vi "test2Dinter.vi"() -> ()   [LabVIEW 2011]
uses:
  finalCalibTypdef.ctl
  <vilib>/gmath/interp.llb/Interpolate 2D (2d X,Y).vi
  <vilib>/Analysis/8numeric.llb/1D Numeric Integration.vi
  <vilib>/Analysis/NI_AALBase.lvlib
  <vilib>/Analysis/1siggen.llb/Ramp Pattern by Samples.vi
  <vilib>/Analysis/NI_AALPro.lvlib
  <vilib>/gmath/NI_Gmath.lvlib
panel:
  out "subarray":dbl[](graph)
  out "time: 2Dinter":u32=126
  out "time: prepare arrays":u32
  in  "final":T1={"X"=array140x256[35840 elements], "xi"=array140x69[9660 elements], "delta momentum"=0.5, "Y"=array92x256[23552 elements], "yi"=array140x69[9660 elements], "angle (Y)"=[-3.7480215406122, -3.6980215406122, -3.6480215406122, -3.5980215406122, -3.5480215406121998, -3.4980215406122, -3.4480215406122, -3.3980215406122, -3.3480215406122, -3.2980215406121998, -3.2480215406122, -3.1980215406122, -3.1480215406122, -3.0980215406122, -3.0480215406121998, -2.9980215406122, -2.9480215406122, -2.8980215406122, -2.8480215406122, -2.7980215406121998, -2.7480215406122, -2.6980215406122, -2.6480215406122, -2.5980215406121996, -2.5480215406121998, -2.4980215406122, -2.4480215406122, -2.3980215406122, -2.3480215406121996, -2.2980215406121998, -2.2480215406122, -2.1980215406122, -2.1480215406122, -2.0980215406121996, -2.0480215406121998, -1.9980215406122, -1.9480215406122, -1.8980215406121999, -1.8480215406121998, -1.7980215406121998, -1.7480215406122, -1.6980215406121997, -1.6480215406121999, -1.5980215406122, -1.5480215406121998, -1.4980215406122, -1.4480215406121997, -1.3980215406121999, -1.3480215406121996, -1.2980215406121998, -1.2480215406122, -1.1980215406121997, -1.1480215406121999, -1.0980215406121996, -1.0480215406121998, -0.9980215406121999, -0.9480215406121997, -0.8980215406121999, -0.8480215406121996, -0.7980215406121998, -0.7480215406121999, -0.6980215406121997, -0.6480215406121999, -0.5980215406121996, -0.5480215406121998, -0.49802154061219994, -0.4480215406121997, -0.39802154061219985, -0.3480215406121996, -0.29802154061219976, -0.24802154061219994, -0.19802154061219968, -0.14802154061219985, -0.09802154061219959, -0.048021540612199765, 0.001978459387800058, 0.051978459387800324, 0.10197845938780015, 0.1519784593878004, 0.20197845938780024, 0.25197845938780006, 0.3019784593877999, 0.3519784593878006, 0.4019784593878004, 0.45197845938780024, 0.5019784593878001, 0.5519784593877999, 0.6019784593878006, 0.6519784593878004, 0.7019784593878002, 0.7519784593878001, 0.8019784593877999, 0.8519784593878006, 0.9019784593878004, 0.9519784593878002, 1.0019784593878, 1.0519784593878008, 1.1019784593878006, 1.1519784593878004, 1.2019784593878002, 1.2519784593878, 1.3019784593878008, 1.3519784593878006, 1.4019784593878004, 1.4519784593878002, 1.5019784593878, 1.5519784593878008, 1.6019784593878006, 1.6519784593878004, 1.7019784593878002, 1.7519784593878, 1.8019784593878008, 1.8519784593878006, 1.9019784593878004, 1.9519784593878002, 2.0019784593878, 2.0519784593878008, 2.1019784593878006, 2.1519784593878004, 2.2019784593878002, 2.2519784593878, 2.3019784593878008, 2.3519784593878006, 2.4019784593878004, 2.4519784593878002, 2.5019784593878, 2.5519784593878008, 2.6019784593878006, 2.6519784593878004, 2.7019784593878002, 2.7519784593878, 2.8019784593878008, 2.8519784593878006, 2.9019784593878004, 2.9519784593878002, 3.0019784593878, 3.0519784593878008, 3.1019784593878006, 3.1519784593878004, 3.2019784593878002], "delta angle"=0.04999999999999982, "scale delta angle"=1.3341308871728326, "intraX"=69.0, "intraY"=140.0, "mask"=array140x69[9660 elements]}
  in  "Y angles 2D":dbl[][](graph)=array92x256[23552 elements]
  in  "Momentum [MeV/C]":dbl[](graph)=[50.07229753265274, 50.15983071443298, 50.24744305307639, 50.335473133793386, 50.42362482327455, 50.512110383361254, 50.60080468664528, 50.68974523698868, 50.77898610800287, 50.86838180578416, 50.95817657226504, 51.04807238565412, 51.138390361009556, 51.22885558514154, 51.31963681309364, 51.41067480417576, 51.50191835219721, 51.593533353084716, 51.68526688034519, 51.777441364408986, 51.869765957355305, 51.962407630762286, 52.05532861013082, 52.148440323478574, 52.24196272933561, 52.33562113373428, 52.429670064721215, 52.52393805106378, 52.61845821707546, 52.71334325025615, 52.8083776798975, 52.90384554844539, 52.999508499681035, 53.09545010289294, 53.19174647851, 53.28820539308308, 53.38510251597625, 53.48220608299536, 53.579579491932385, 53.677325478650495, 53.77524407497087, 53.87356454114524, 53.97213509708919, 54.07092947555539, 54.17015652080565, 54.269570248674576, 54.36932324018744, 54.46941123347271, 54.56969420713886, 54.67041102722302, 54.77137308543024, 54.87257300044643, 54.974216610337685, 55.07606355335658, 55.178218731599664, 55.28075162708607, 55.383497615374985, 55.48661882716664, 55.59006868597277, 55.69374082051916, 55.79784018182734, 55.90223156342043, 56.00684549505606, 56.111873606754635, 56.21720302119806, 56.32283918208316, 56.42882890219444, 56.5351236728704, 56.641720134138744, 56.748684625045605, 56.855953718041384, 56.963538804395505, 57.07149018048698, 57.1797524193871, 57.28834570048473, 57.397296090985385, 57.50656005590199, 57.616172858663234, 57.7261282182496, 57.83640050845812, 57.94704953896948, 58.05802395807821, 58.16933872771148, 58.281018950382276, 58.393019385067475, 58.50539236287636, 58.61810188547397, 58.731156613509306, 58.844584735455136, 58.95833890016895, 59.07248879093084, 59.18696647546072, 59.30181925309975, 59.417024114353715, 59.53258299516336, 59.64851910190262, 59.76479881890396, 59.88148018668999, 59.9984946345451, 60.115921847826904, 60.23368516435314, 60.35185067203749, 60.470364539014994, 60.58927639342781, 60.70854834588829, 60.8282217835343, 60.94825921065038, 61.06870460119095, 61.18951111605114, 61.310724517923916, 61.43229968923823, 61.554292936903096, 61.67664895324813, 61.799436232216266, 61.922589641352786, 62.04618162330728, 62.17014251711384, 62.29452558712144, 62.41929351908275, 62.54446961953862, 62.67006038580525, 62.7960388070786, 62.92246671292553, 63.04927783564081, 63.176524732148735, 63.304179330384684, 63.43223718780839, 63.560740627474246, 63.689640295677854, 63.81898202265973, 63.94874959300494, 64.07892098001717, 64.20955602995856, 64.34059773887691, 64.47206231218102, 64.60397897467172, 64.73631237640821, 64.869085738597, 65.00231471477268, 65.13596573408442, 65.27006683532953, 65.40462738222232, 65.53962005497071, 65.67506033230055, 65.8109815987919, 65.9473433427755, 66.0841535752014, 66.22144522937742, 66.35918942385068, 66.49737914455044, 66.63602368841578, 66.7751474034366, 66.91472762039646, 67.05476469204305, 67.19527658421696, 67.33628142329019, 67.47775433008199, 67.61969559362808, 67.76210633768139, 67.90501441704042, 68.04840416594494, 68.19226957401172, 68.33661620544575, 68.48144943209485, 68.62679493465447, 68.77262969523863, 68.91895730915441, 69.06577899650894, 69.21310202770283, 69.36092815635924, 69.50927035473094, 69.65811068326026, 69.80744438410392, 69.9572688425338, 70.10759120897865, 70.25841815946569, 70.4097512757638, 70.56160058811538, 70.71397754166274, 70.86686942159963, 71.02027152856012, 71.17418729848787, 71.32861278943483, 71.48355948930313, 71.63903383298718, 71.79503909451408, 71.95157896275194, 72.10865976498366, 72.26627835863347, 72.42443773423045, 72.58313719524446, 72.74237809740015, 72.90216284371118, 73.06249307935462, 73.22337570366312, 73.38481299401033, 73.54681679847542, 73.70938657108235, 73.87252626016662, 74.03623956556689, 74.20052907315498, 74.36539661252398, 74.53084771684584, 74.6968830777154, 74.86350384169735, 75.03070688990859, 75.19849228216307, 75.36687898015636, 75.53585900252442, 75.70544362170186, 75.87563942077512, 76.04645285122083, 76.21787961399053, 76.38991264403143, 76.56255744104838, 76.73582111277462, 76.9096873341793, 77.08416070831274, 77.25925052021022, 77.4349600453981, 77.6113063980163, 77.78827696200767, 77.9658595260864, 78.14405451011176, 78.32286883536608, 78.50233423633921, 78.68243479312856, 78.8631773205512, 79.0445771403343, 79.22665527344569, 79.40938326412468, 79.59275150859004, 79.77678280996797, 79.96146342460078, 80.14678490571335, 80.3327747387059, 80.51944409828232, 80.70678449184061, 80.89483312815786, 81.08358530541098, 81.27300980796292, 81.463137571359, 81.65394598409715, 81.84543408487188, 82.03763762101902, 82.23053281769182, 82.42416900544262, 82.61852659219059, 82.81361926820861, 83.00944812670377, 83.20598132803654, 83.40325366033011, 83.6012275391606, 83.79997131222892, 83.99943721084946, 84.19970193525548]
  in  "pixel angle (y)":dbl[](array[numeric])=[0.037477582207811125, 0.0375378103280183, 0.03759835324988168, 0.037638239676906486, 0.03767220925926772, 0.037689747456214555, 0.037718124937573545, 0.037759339175450615, 0.037815945617947995, 0.03788063743518453, 0.037925600705336834, 0.03796557132360937, 0.0379840699612592, 0.03800781476200766, 0.03804282848571206, 0.03808205383420604, 0.038124687047283425, 0.03819497257668394, 0.03827047431284569, 0.03831511839702091, 0.03834959008082911, 0.038362398521621585, 0.03839429519350118, 0.03843930535194785, 0.038506475559157566, 0.03857307729220705, 0.038620070814944035, 0.03866676181810502, 0.0387130848375811, 0.03873601391808348, 0.03875484132448539, 0.03880297443490419, 0.03886161595012056, 0.03893532872686465, 0.03881951069724796, 0.038611566223731374, 0.038105163864268106, 0.03769554724778958, 0.03740223373517817, 0.03723603496248856, 0.037173529161227875, 0.03749521823198995, 0.03783880798538115, 0.03820360723024477, 0.038739908755063765, 0.03919553366910764, 0.039389798714018424, 0.03953215344479871, 0.03964512210299738, 0.03969861147758047, 0.03976617071201567, 0.03984752086655404, 0.03990445098286168, 0.03995783288040166, 0.04000815111780023, 0.04004296007757376, 0.04007772601145543, 0.04012660954541183, 0.04020430873594673, 0.04029042274207045, 0.040339384000090406, 0.04039344990701764, 0.04044723736216941, 0.040462083471605036, 0.040551826962865384, 0.04057158550151761, 0.04064707182832961, 0.04069310897748229, 0.040726185871045435, 0.0407104047486137, 0.040722698074851925, 0.040790994765831104, 0.040786483184387635, 0.040900331433328066, 0.04100957841477542, 0.04113275717285748, 0.04128943624065327, 0.041383986129591356, 0.04152035652895744, 0.04158841056385747, 0.041693110815272556, 0.04176647471980758, 0.041808109547457964, 0.041896373749087015, 0.041945596201376605, 0.04203752144656966, 0.042096929899642394, 0.04216377175264231, 0.04221267837449374, 0.04225164716353927, 0.04233033219068084, 0.04240479044280577, 0.0424280109007416, 0.04252130522978519, 0.04255646064460216, 0.04262159712046446, 0.04271106684539846, 0.042726953841267706, 0.042834365027920374, 0.04285980067144029, 0.04290407847360533, 0.04298148359330201, 0.043059352930560964, 0.04310666304059418, 0.04318186470763455, 0.04321124753836594, 0.04326638956928416, 0.04336841907624626, 0.043372840226511486, 0.04344502754224136, 0.043458805969808625, 0.04350176453092871, 0.04354504692756502, 0.043572282445234374, 0.043719886246918596, 0.04377506306562891, 0.0438307216429467, 0.043882255177807514, 0.043967069555529224, 0.04404340617312178, 0.044087710081034515, 0.04422154778325681, 0.04424178336968342, 0.04425229311880168, 0.044328392796142854, 0.04440326745130848, 0.04447921973832866, 0.04449440271083517, 0.0445909980356023, 0.04465122004116054, 0.04469582940733911, 0.044746207718220174, 0.044675726002842364, 0.04267205785741442, 0.04276641846475699, 0.04280525728079379, 0.04285689437155202, 0.042923903830319854, 0.04301110520013367, 0.0431323830019876, 0.04316545752017941, 0.04328575986704131, 0.043384775227001564, 0.04349267378173057, 0.04355348288319274, 0.043604651859098995, 0.043716347210854205, 0.04378821118055596, 0.04386448742162739, 0.04399794933329327, 0.04404503831307389, 0.04421272483161148, 0.044331415250278665, 0.04440921929214469, 0.04454672370056835, 0.04460184505873057, 0.04466448019056487, 0.04475018057724128, 0.04484458912204318, 0.044920986274926945, 0.045002289062931904, 0.045097118158317455, 0.04518240711607863, 0.045269624867765396, 0.04541703071251877, 0.04550795280628246, 0.04559946882095624, 0.04571174005768977, 0.0460750366911433, 0.04639562647607986, 0.04674801712470383, 0.04710979552536287, 0.047363521515647794, 0.04741983739378383, 0.04732957065712525, 0.047199255919237446, 0.04702192063132577, 0.04689077900955041, 0.04721790956291122, 0.04754662503244337, 0.04779302473044378, 0.04818681974992477, 0.04858485464933235, 0.04869299591718263, 0.048584550402762744, 0.0484764930169296, 0.04835834443169048, 0.04828719469900186, 0.048222766428404916, 0.04834188706300746, 0.04846143489496384, 0.04857102710814599, 0.04868653104243684, 0.04880619805934796, 0.04893075858982508, 0.04908427889763241, 0.049511031973531044, 0.049898237974339496, 0.05040624016531754, 0.050837732267569075, 0.05134015949012785, 0.0516218346028756, 0.05178360005226867, 0.05194105378254242, 0.05214945752433647, 0.052362654325496354, 0.05255736775078291, 0.05271697114435879, 0.052902655552384936, 0.05345104909708188, 0.05400078856621423, 0.05457402723638789, 0.05525483903273678, 0.05589234596637011, 0.056344461115130355, 0.05660466064617305, 0.05684739692395777, 0.056939091390825536, 0.057216581293874316, 0.05752631629729546, 0.05776594597871566, 0.057970210025959985, 0.05834620444709129, 0.059095734294158916, 0.05966843750713058, 0.060504562685601664, 0.06104390929579467, 0.06184660565948633, 0.06229432111910379, 0.06285675616055271, 0.06335993292100976, 0.0640103781230761, 0.06494640922743135, 0.06537375904368167, 0.06452970332711605, 0.06398947667297139, 0.06318949092368346, 0.06310561739014162, 0.06273982627858529, 0.06317953539335003, 0.064788318139689, 0.0670660575425553, 0.06825261980428583, 0.06928919838614656, 0.07047135756226576, 0.07108681736337749, 0.07212300303227219, 0.07274371033405448, 0.07331974443237226, 0.07396837480214184, 0.07437897672000632, 0.07495723436598267, 0.07528920281146867, 0.07587775203900965, 0.0762276605751895, 0.07649023552269796]
  out "time: spectra":u32=1
  out "spec cluster 2":cluster{"Momentum [MeV/C]":dbl[], dbl[]}(graph)={"Momentum [MeV/C]"=[50.07229753265274, 50.57229753265274, 51.07229753265274, 51.57229753265274, 52.07229753265274, 52.57229753265274, 53.07229753265274, 53.57229753265274, 54.07229753265274, 54.57229753265274, 55.07229753265274, 55.57229753265274, 56.07229753265274, 56.57229753265274, 57.07229753265274, 57.57229753265274, 58.07229753265274, 58.57229753265274, 59.07229753265274, 59.57229753265274, 60.07229753265274, 60.57229753265274, 61.07229753265274, 61.57229753265274, 62.07229753265274, 62.57229753265274, 63.07229753265274, 63.57229753265274, 64.07229753265274, 64.57229753265274, 65.07229753265274, 65.57229753265274, 66.07229753265274, 66.57229753265274, 67.07229753265274, 67.57229753265274, 68.07229753265274, 68.57229753265274, 69.07229753265274, 69.57229753265274, 70.07229753265274, 70.57229753265274, 71.07229753265274, 71.57229753265274, 72.07229753265274, 72.57229753265274, 73.07229753265274, 73.57229753265274, 74.07229753265274, 74.57229753265274, 75.07229753265274, 75.57229753265274, 76.07229753265274, 76.57229753265274, 77.07229753265274, 77.57229753265274, 78.07229753265274, 78.57229753265274, 79.07229753265274, 79.57229753265274, 80.07229753265274, 80.57229753265274, 81.07229753265274, 81.57229753265274, 82.07229753265274, 82.57229753265274, 83.07229753265274, 83.57229753265274, 84.07229753265274], [0.0867981540222726, 0.08261634745549262, 0.15780243233786856, 0.14775796013035777, 0.05263053391121891, 0.053052912294376156, 0.15191318594308015, 0.14981983430136114, 0.11700139206762095, 0.13155222887076734, 0.1684249055215002, 0.16857865833690094, 0.14176424686395364, 0.14427921628046295, 0.1644688231907754, 0.1635416016001087, 0.1420908968440197, 0.14020609014657043, 0.1588669769760078, 0.15589370121820792, 0.14174948409773352, 0.13341276225310042, 0.13536702340099901, 0.14916877693013172, 0.14718055167799698, 0.12846317488550774, 0.12676970679561064, 0.12937916674428734, 0.13973463531757968, 0.13218113303417095, 0.11053750184758489, 0.10576539321438339, 0.10038686906156509, 0.12463763630849774, 0.12106677338062412, 0.12028186596589945, 0.09139884919877436, 0.09412084211729885, 0.12365896282614211, 0.12893346320853483, 0.13058812446128448, 0.10610796495898847, 0.10366759807927937, 0.10497898421031235, 0.12419714648561285, 0.13205036294523848, 0.13253036025692783, 0.1309733623420704, 0.1137779761530524, 0.11728841296657326, 0.12239930144646781, 0.14675371437352117, 0.15014047187903135, 0.15234650208833272, 0.13443316248670253, 0.12377935992042939, 0.12145373556854189, 0.1416095768605585, 0.16143985441865993, 0.1655396857388431, 0.16905287974194014, 0.13483627511386545, 0.12806962985094095, 0.13850098246313058, 0.14688829788141392, 0.18928965954454857, 0.19215368111241415, 0.19521128738469867, 0.20641294822426734]}
  out "charge (spectra)":dbl=4.5665602092068625 format="%0.4f"
  out "charge (YSum)":dbl=4.639584559364366 format="%0.4f"
  out "Sum Y":cluster{"Ramp Pattern":dbl[], dbl[]}={"Ramp Pattern"=[-3.7480215406122, -3.6980215406122, -3.6480215406122, -3.5980215406122, -3.5480215406121998, -3.4980215406122, -3.4480215406122, -3.3980215406122, -3.3480215406122, -3.2980215406121998, -3.2480215406122, -3.1980215406122, -3.1480215406122, -3.0980215406122, -3.0480215406121998, -2.9980215406122, -2.9480215406122, -2.8980215406122, -2.8480215406122, -2.7980215406121998, -2.7480215406122, -2.6980215406122, -2.6480215406122, -2.5980215406121996, -2.5480215406121998, -2.4980215406122, -2.4480215406122, -2.3980215406122, -2.3480215406121996, -2.2980215406121998, -2.2480215406122, -2.1980215406122, -2.1480215406122, -2.0980215406121996, -2.0480215406121998, -1.9980215406122, -1.9480215406122, -1.8980215406121999, -1.8480215406121998, -1.7980215406121998, -1.7480215406122, -1.6980215406121997, -1.6480215406121999, -1.5980215406122, -1.5480215406121998, -1.4980215406122, -1.4480215406121997, -1.3980215406121999, -1.3480215406121996, -1.2980215406121998, -1.2480215406122, -1.1980215406121997, -1.1480215406121999, -1.0980215406121996, -1.0480215406121998, -0.9980215406121999, -0.9480215406121997, -0.8980215406121999, -0.8480215406121996, -0.7980215406121998, -0.7480215406121999, -0.6980215406121997, -0.6480215406121999, -0.5980215406121996, -0.5480215406121998, -0.49802154061219994, -0.4480215406121997, -0.39802154061219985, -0.3480215406121996, -0.29802154061219976, -0.24802154061219994, -0.19802154061219968, -0.14802154061219985, -0.09802154061219959, -0.048021540612199765, 0.001978459387800058, 0.051978459387800324, 0.10197845938780015, 0.1519784593878004, 0.20197845938780024, 0.25197845938780006, 0.3019784593877999, 0.3519784593878006, 0.4019784593878004, 0.45197845938780024, 0.5019784593878001, 0.5519784593877999, 0.6019784593878006, 0.6519784593878004, 0.7019784593878002, 0.7519784593878001, 0.8019784593877999, 0.8519784593878006, 0.9019784593878004, 0.9519784593878002, 1.0019784593878, 1.0519784593878008, 1.1019784593878006, 1.1519784593878004, 1.2019784593878002, 1.2519784593878, 1.3019784593878008, 1.3519784593878006, 1.4019784593878004, 1.4519784593878002, 1.5019784593878, 1.5519784593878008, 1.6019784593878006, 1.6519784593878004, 1.7019784593878002, 1.7519784593878, 1.8019784593878008, 1.8519784593878006, 1.9019784593878004, 1.9519784593878002, 2.0019784593878, 2.0519784593878008, 2.1019784593878006, 2.1519784593878004, 2.2019784593878002, 2.2519784593878, 2.3019784593878008, 2.3519784593878006, 2.4019784593878004, 2.4519784593878002, 2.5019784593878, 2.5519784593878008, 2.6019784593878006, 2.6519784593878004, 2.7019784593878002, 2.7519784593878, 2.8019784593878008, 2.8519784593878006, 2.9019784593878004, 2.9519784593878002, 3.0019784593878, 3.0519784593878008, 3.1019784593878006, 3.1519784593878004, 3.2019784593878002], [0.011137016165256157, 0.021829482575962254, 0.03253936074405018, 0.03253936074405018, 0.04311640649190382, 0.04311640649190382, 0.05396432999147681, 0.05396432999147681, 0.05396432999147681, 0.0648405149308176, 0.0648405149308176, 0.07519709540305819, 0.08532238926169682, 0.10645960013879904, 0.11646552616110853, 0.1262931972965455, 0.1262931972965455, 0.13613073955062374, 0.14616184635933333, 0.1568268520872908, 0.16764674670326793, 0.1792333420896368, 0.1792333420896368, 0.19119255194621682, 0.21580323036808718, 0.22798757479306148, 0.24004934637789171, 0.27425739243614305, 0.2954593954326747, 0.3268444217371545, 0.33699626234794267, 0.3972438893400589, 0.4975079821041705, 0.5784550978937094, 0.6237641671768127, 0.670223308632034, 0.6972386282522536, 0.7194304027948516, 0.7614949581566398, 0.7750502096335162, 0.8081105417562462, 0.8400022408477874, 0.8625280417911433, 0.8842068672698414, 0.9042665147796451, 0.9307604876664245, 1.141986935321149, 1.1459565922804242, 1.1499446962467175, 1.1534926992504548, 1.157688284154065, 1.1602617774340027, 1.1628196339295893, 1.0532823804226565, 1.0068490061377193, 1.0018659739534326, 1.0077449998924777, 1.0106962243007982, 1.0201814437681154, 1.1327018238729718, 1.1841597444446181, 1.1898496190570238, 1.1917683993566488, 1.1944768150871825, 1.197472826548403, 1.196932235338961, 1.1761955574199705, 1.0340587513385475, 1.0326774256268136, 1.0333844213877457, 1.0333800781324616, 1.0365329736868745, 1.0533459332692046, 1.2020056041761717, 1.2060281105825565, 1.2050317606479317, 1.204201827833067, 1.2043812850997597, 1.2046266645753132, 1.1996280056100217, 1.0677778229501242, 1.0209979917006726, 1.0152144652017994, 1.0150612256540354, 1.0176812530801653, 1.024219078901479, 1.150812963763347, 1.2064688058325819, 1.208526307739713, 1.2098977578471666, 1.2103459979931248, 1.2124905744228602, 1.2136908075909367, 1.1858763420838527, 1.0053181621971135, 0.9979875683723081, 0.9933271834735534, 0.9872596918513727, 0.9810110365998367, 0.9985706652221166, 1.2003841515450748, 1.2036401493895261, 1.1982963556918365, 1.1922389934162032, 1.1863304015351999, 1.1669414647412235, 1.1581835128027165, 1.017484351991429, 0.9006904091068436, 0.8586545614337409, 0.7663944573911133, 0.6290660218141425, 0.5007457951411629, 0.4280535100713805, 0.4099891022028317, 0.38164291917095694, 0.29668556124489337, 0.2797331706247183, 0.2715140650224642, 0.26328795499237434, 0.23670749597480242, 0.21926816308825772, 0.21926816308825772, 0.1883408228071427, 0.1707249762001949, 0.1707249762001949, 0.15632749156797304, 0.14855651092515887, 0.12097184081735882, 0.10366193619417946, 0.08636660795112303, 0.08636660795112303, 0.08636660795112303, 0.0784992419374238, 0.0784992419374238, 0.06971613723795841, 0.06971613723795841, 0.03515066658752093, 0.017933506702217872, 0.0]}
  out "Array":dbl[][](array[numeric])
  out "charge (sum)":dbl=4.639862984768497
  out "charge density":dbl[][](array[numeric])
  out "Z 2":dbl[][](graph)
  out "size(s)":i32[](array[numeric])=[140, 69]
  out "size(s) 2":i32[](array[numeric])=[140, 69]
  in  "empty image":bool
  in  "Z":dbl[][](graph)=array92x256[23552 elements]
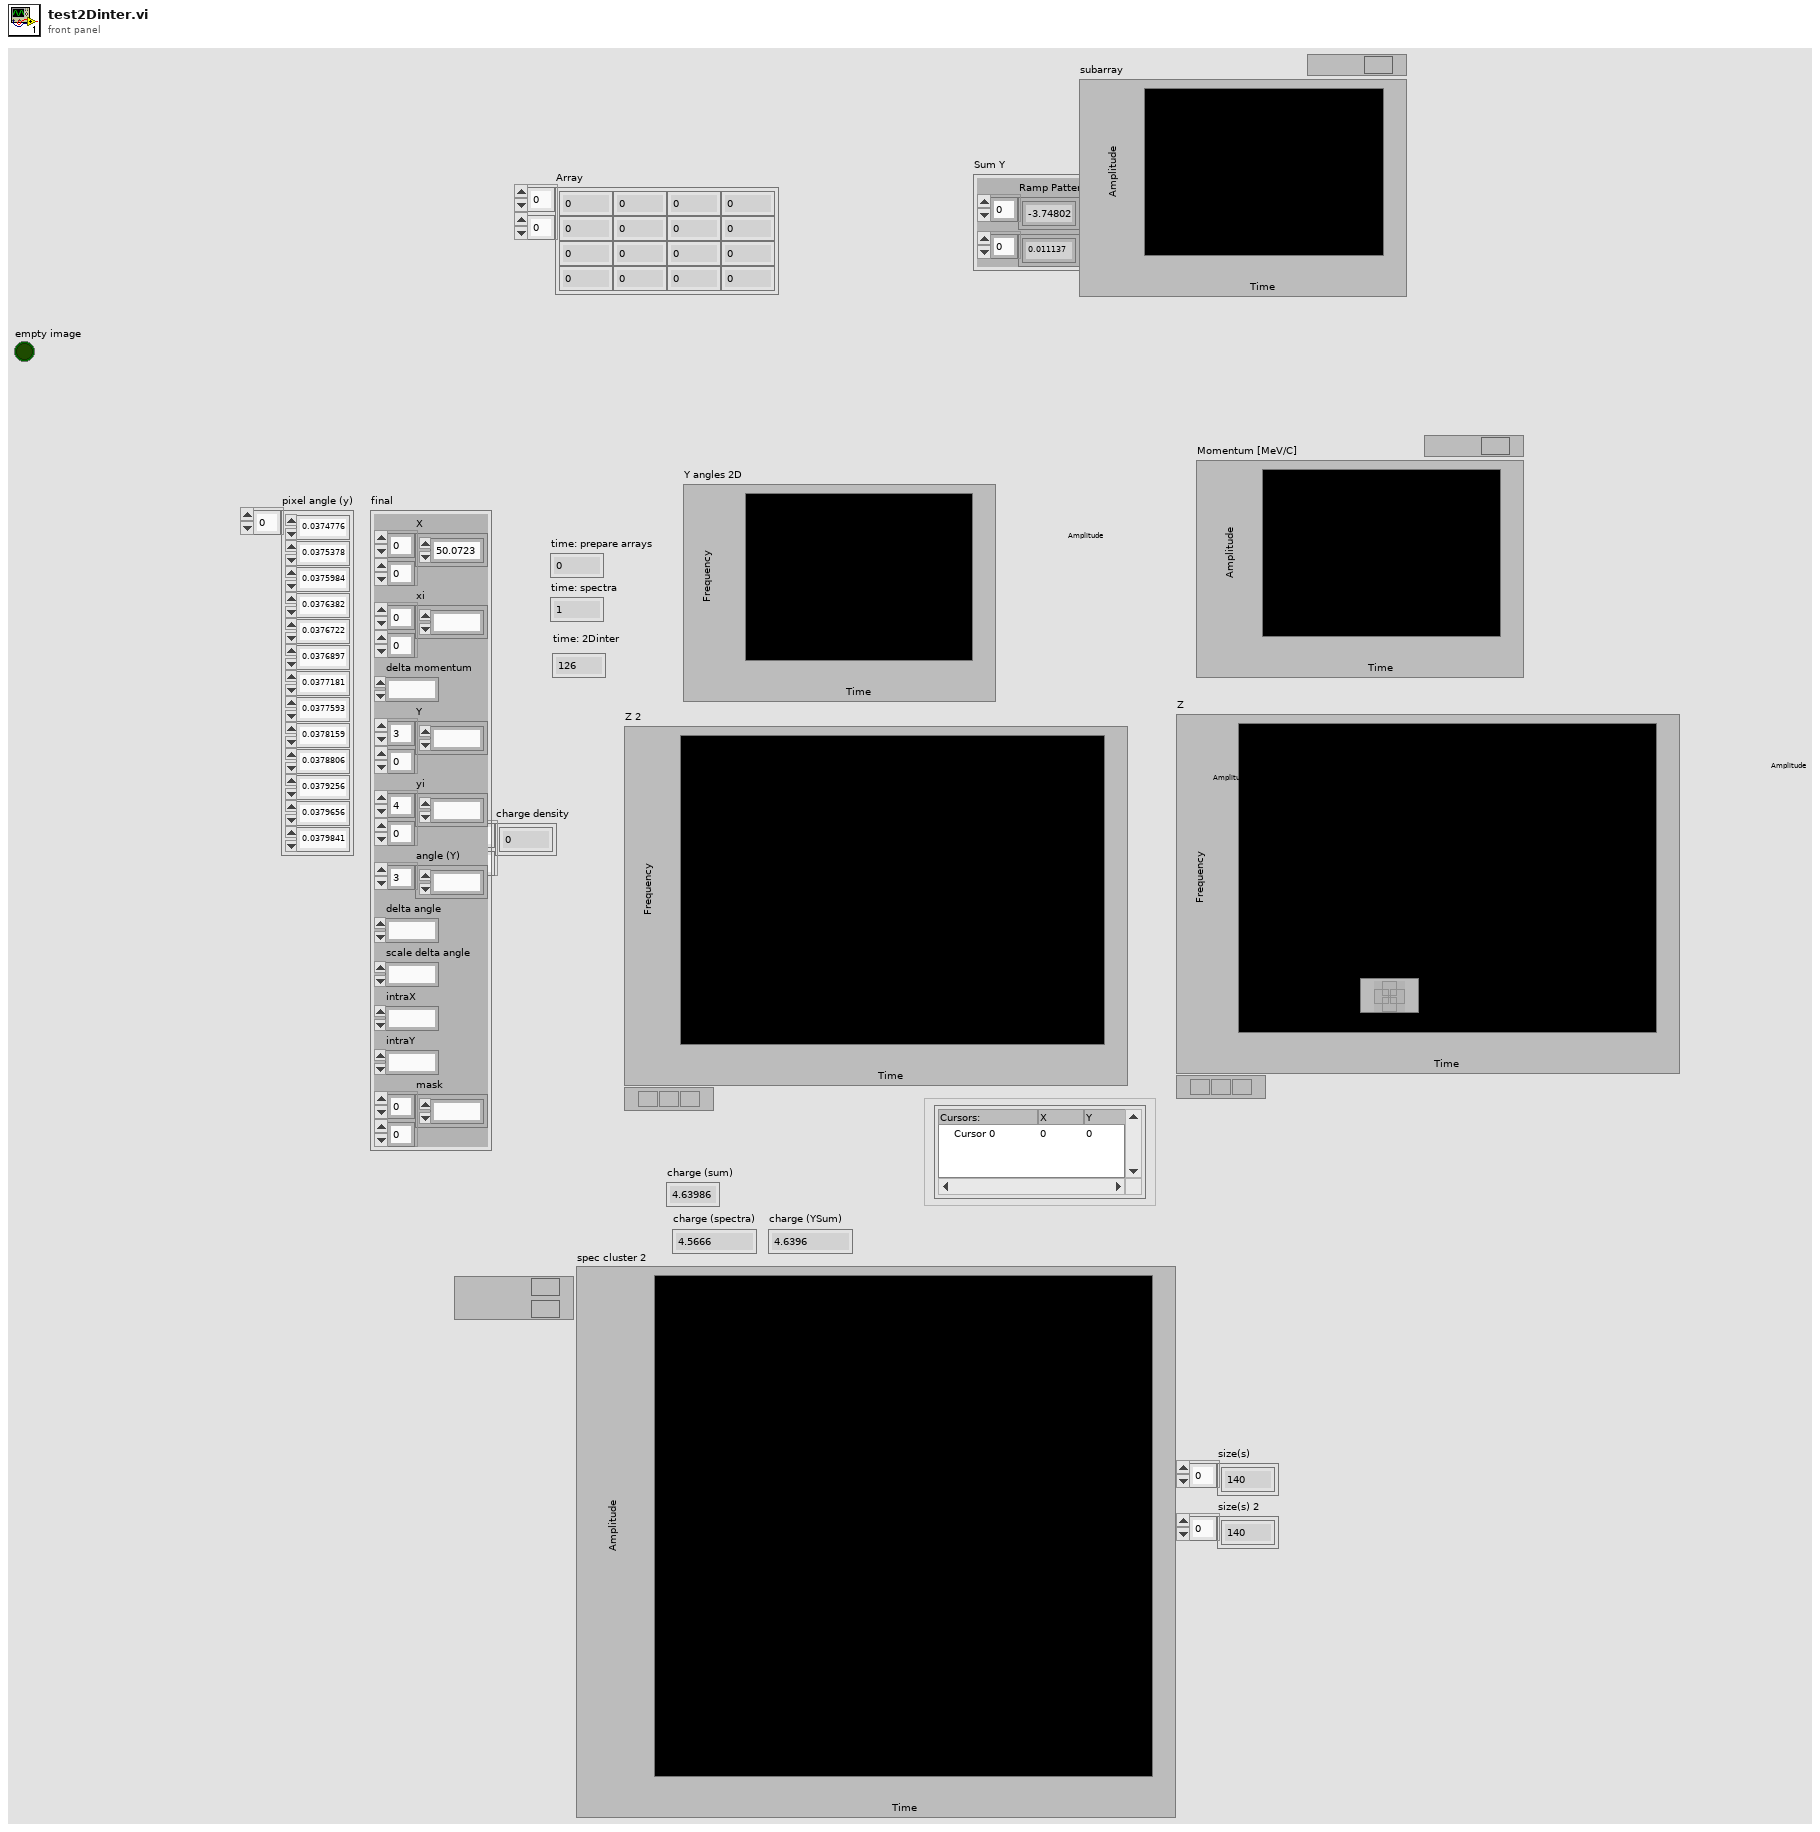
[diagram p1: front panel]
types:
  T1 = typedef "finalCalibTypdef.ctl" = cluster{"X":dbl[][], "xi":dbl[][], "delta momentum":dbl, "Y":dbl[][], "yi":dbl[][], "angle (Y)":dbl[], "delta angle":dbl, "scale delta angle":dbl, "intraX":dbl, "intraY":dbl, "mask":dbl[][]}
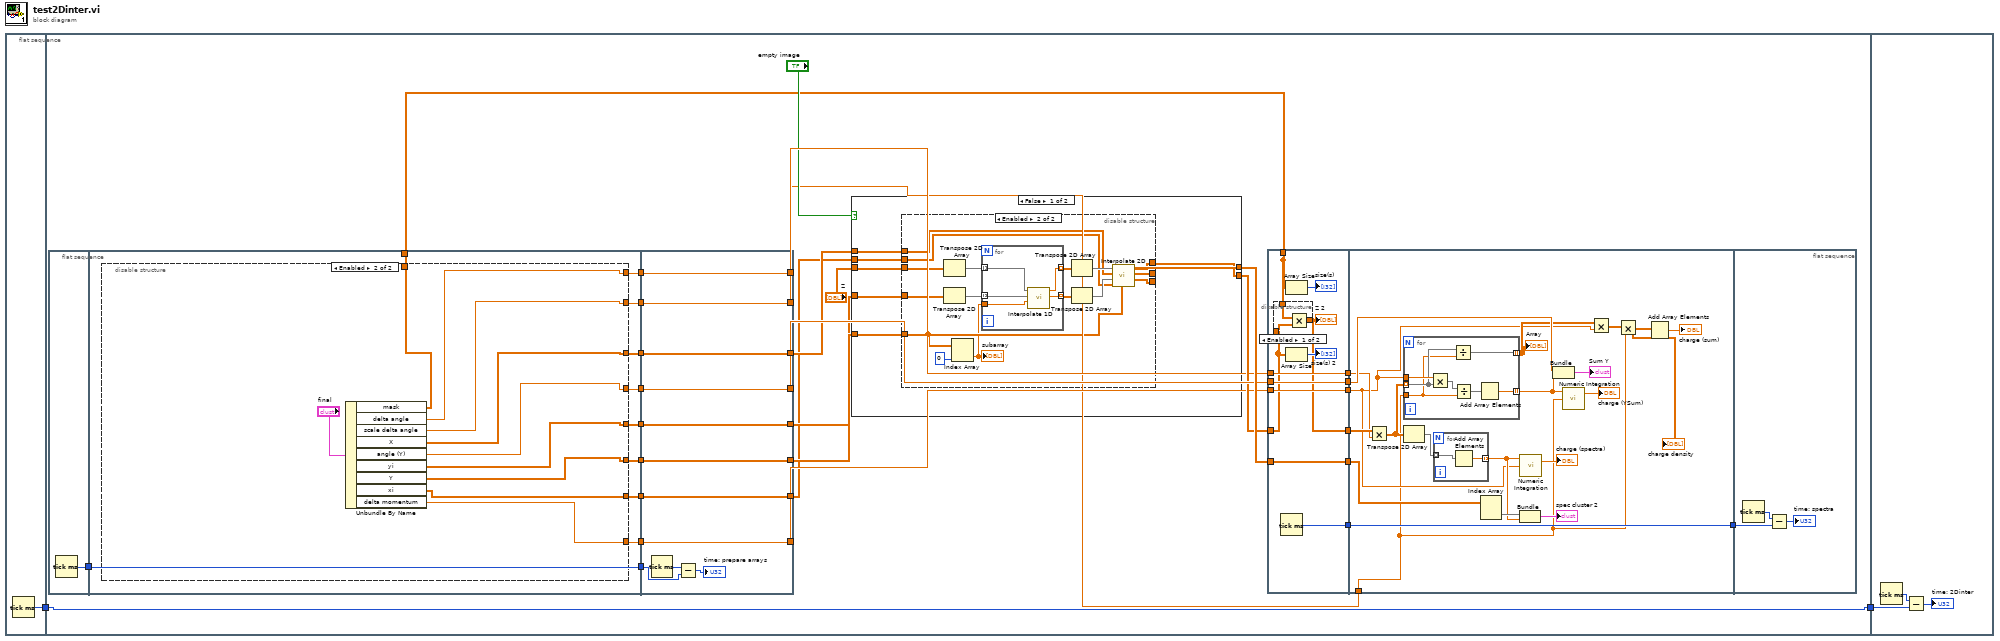
[diagram p0: block diagram]
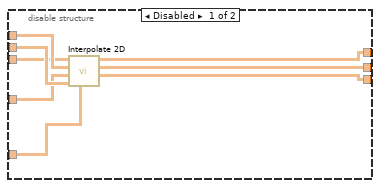
[diagram p2: hidden frame]
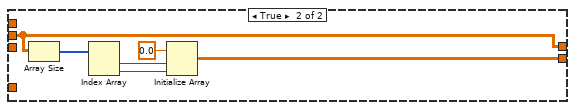
[diagram p3: hidden frame]
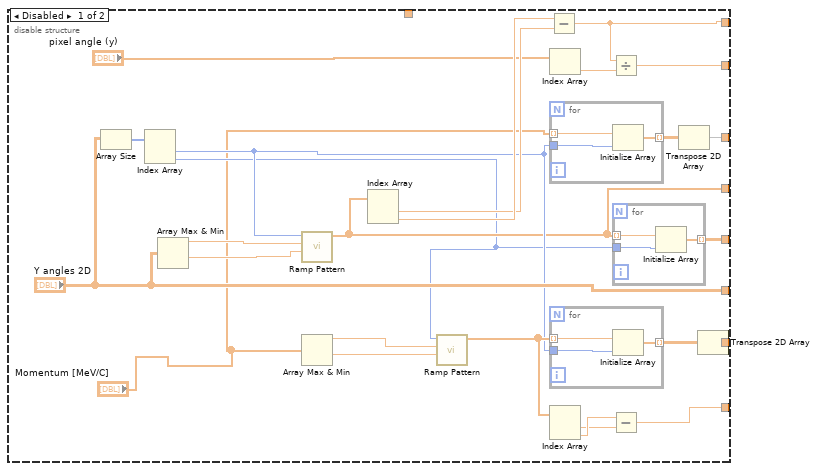
[diagram p5: hidden frame]
diagram:
  n1 = flat-sequence {
    tunnel: [w3] -> w2
    tunnel: w2 -> [w34]
    tunnel: [w34] -> w1
    tunnel: w1 -> [w191]
    frame #0 {
      n2 = Tick Count (ms)() -> (millisecond timer value=w3:u32)
    }
    frame #1 {
      n3 = flat-sequence {
        tunnel: [w124] -> w22
        tunnel: [w134] -> w29
        tunnel: [w133] -> w28
        tunnel: [w132] -> w27
        tunnel: [w126] -> w26
        tunnel: [w131] -> w25
        tunnel: [w130] -> w24
        tunnel: [w129] -> w23
        tunnel: w22 -> [w128]
        tunnel: [w128] -> w21
        tunnel: [w127] -> w11
        tunnel: [w125] -> w4
        tunnel: [w184] -> w7
        tunnel: [w185] -> w6
        tunnel: [w186] -> w30
        tunnel: [w180] -> w32
        tunnel: [w187] -> w13
        tunnel: [w188] -> w5
        tunnel: [w189] -> w8
        tunnel: w29 -> [w189]
        tunnel: w28 -> [w188]
        tunnel: w27 -> [w187]
        tunnel: w26 -> [w180]
        tunnel: w25 -> [w186]
        tunnel: w24 -> [w185]
        tunnel: w23 -> [w184]
        tunnel: w21 -> [w182]
        tunnel: [w179] -> w10
        tunnel: w11 -> [w179]
        frame #0 {
          n4 = Tick Count (ms)() -> (millisecond timer value=w124:u32)
        }
        frame #1 {
          n5 = disable-structure shown="Enabled" {
            disable-tunnel: [w157 w175] -> w134
            disable-tunnel: [w153 w171] -> w133
            disable-tunnel: [w147 w170] -> w132
            disable-tunnel: [w146 w176] -> w131
            disable-tunnel: ["Y angles 2D" w172] -> w130
            disable-tunnel: [w143 w173] -> w129
            disable-tunnel: [w139 w177] -> w127
            disable-tunnel: [w137 w174] -> w126
            disable-tunnel: [_ w169] -> w125
            frame Disabled {
              n6 = Array Size(array="Y angles 2D") -> (size(s)=w159:i32[])
              n7 = Index Array(array=w159) -> (element #1=w138:i32, element #2=w136:i32)  [unwired: 2 in]
              n8 = Array Max & Min(array="Y angles 2D") -> (max value=w140:dbl, min value=w141:dbl)  [unwired: 2 out]
              n9 = call-poly <vilib>:"Ramp Pattern.vi"("start"=w141, "end"=w140, "samples"=w138) -> ("Ramp Pattern"=w137:dbl[])  [unwired: 7 in, 1 out]
              n10 = Array Max & Min(array="Momentum [MeV/C]") -> (max value=w156:dbl, min value=w155:dbl)  [unwired: 2 out]
              n11 = Index Array(array=w137) -> (element #1=w151:dbl, element #2=w152:dbl)  [unwired: 2 in]
              n12 = call-poly <vilib>:"Ramp Pattern.vi"("start"=w155, "end"=w156, "samples"=w136) -> ("Ramp Pattern"=w150:dbl[])  [unwired: 7 in, 1 out]
              n13 = Subtract(x=w152, y=w151) -> (x-y=w139:dbl)
              n14 = Index Array(array="pixel angle (y)") -> (element=w145:dbl)  [unwired: 1 in]
              n15 = for {
                tunnel: "Momentum [MeV/C]" -> [w168] mode=indexing
                tunnel: w138 -> [w167]
                tunnel: [w166] -> w158 mode=indexing
                n16 = Initialize Array(w168, w167) -> (w166:dbl[])
              }
              n17 = for {
                tunnel: w150 -> [w165] mode=indexing
                tunnel: w138 -> [w164]
                tunnel: [w163] -> w154 mode=indexing
                n18 = Initialize Array(w165, w164) -> (w163:dbl[])
              }
              n19 = Index Array(array=w150) -> (element #1=w148:dbl, element #2=w149:dbl)  [unwired: 2 in]
              n20 = Divide(x=w139, y=w145) -> (x/y=w146:dbl)
              n21 = Subtract(x=w149, y=w148) -> (x-y=w147:dbl)
              n22 = for {
                tunnel: w137 -> [w162] mode=indexing
                tunnel: w136 -> [w161]
                tunnel: [w160] -> w143 mode=indexing
                n23 = Initialize Array(w162, w161) -> (w160:dbl[])
              }
              n24 = Transpose 2D Array(2D array=w158) -> (transposed array=w157:dbl[][])
              n25 = Transpose 2D Array(2D array=w154) -> (transposed array=w153:dbl[][])
            }
            frame Enabled {
              n26 = Unbundle By Name("final") -> ("mask"=w169:dbl[][], "delta angle"=w177:dbl, "scale delta angle"=w176:dbl, "X"=w175:dbl[][], "angle (Y)"=w174:dbl[], "yi"=w173:dbl[][], "Y"=w172:dbl[][], "xi"=w171:dbl[][], "delta momentum"=w170:dbl)
            }
          }
        }
        frame #2 {
          n27 = Tick Count (ms)() -> (millisecond timer value=w183:u32)
          n28 = Subtract(x=w183, y=w182) -> (x-y=→"time: prepare arrays":u32)
        }
      }
      n29 = case shown="False" "empty image" {
        tunnel: w8 -> [w41 _]
        tunnel: [w40 w76] -> w33
        tunnel: w5 -> [w39 w76]
        tunnel: "Z" -> [w38 _]
        tunnel: [w37 w72] -> w31
        tunnel: w6 -> [w36 _]
        tunnel: w7 -> [w35 _]
        frame False {
          n30 = disable-structure shown="Enabled" {
            disable-tunnel: w41 -> [w50 w62]
            disable-tunnel: [w49 w59] -> w40
            disable-tunnel: w39 -> [w48 w61]
            disable-tunnel: w38 -> [w47 w57]
            disable-tunnel: [w46 w60] -> w37
            disable-tunnel: w36 -> [w45 w54]
            disable-tunnel: [w43 w58] -> _
            disable-tunnel: w35 -> [w42 w52]
            frame Disabled {
              n31 = call-poly <vilib>:"Interpolate 2D.vi"("yi"=w42, "xi"=w48, "Y"=w45, "X"=w50, "Z"=w47) -> ("error"=w44:i32, "yi used"=w43:dbl[][], "xi used"=w49:dbl[][], "zi"=w46:dbl[][])  [unwired: 3 in]
            }
            frame Enabled {
              n32 = Transpose 2D Array(2D array=w57) -> (transposed array=w55:dbl[][])
              n33 = Transpose 2D Array(2D array=w54) -> (transposed array=w53:dbl[][])
              n34 = Index Array(array=w52, index (col)=0 ("disabled index (col)")) -> (element=w51:dbl[])  [unwired: 1 in]
              "subarray" <- w51
              n35 = for {
                tunnel: w55 -> [w71] mode=indexing
                tunnel: w53 -> [w70] mode=indexing
                tunnel: w51 -> [w69]
                tunnel: [w68] -> w66 mode=indexing
                tunnel: [w67] -> w64 mode=indexing
                n36 = call <vilib>:"Interpolate 1D.vi"("xi"=w69, "X"=w70, "Y"=w71) -> ("xi used"=w67:dbl[], "yi"=w68:dbl[])  [unwired: 6 in, 1 out]
              }
              n37 = Transpose 2D Array(2D array=w66) -> (transposed array=w65:dbl[][])
              n38 = Transpose 2D Array(2D array=w64) -> (transposed array=w63:dbl[][])
              n39 = call-poly <vilib>:"Interpolate 2D.vi"("yi"=w52, "xi"=w61, "Y"=w63, "X"=w62, "Z"=w65) -> ("yi used"=w58:dbl[][], "xi used"=w59:dbl[][], "zi"=w60:dbl[][])  [unwired: 3 in, 1 out]
            }
          }
        }
        frame True {
          n40 = Array Size(array=w76) -> (size(s)=w75:i32[])
          n41 = Index Array(array=w75) -> (element #1=w74:i32, element #2=w73:i32)  [unwired: 2 in]
          n42 = Initialize Array(0.0 ("element"), w74, w73) -> (w72:dbl[][])
        }
      }
      n43 = flat-sequence {
        tunnel: w30 -> [w86]
        tunnel: w31 -> [w83]
        tunnel: w32 -> [w87]
        tunnel: w33 -> [w78]
        tunnel: [w78] -> w20
        tunnel: [w87] -> w19
        tunnel: [w79] -> w18
        tunnel: [w86] -> w17
        tunnel: [w85] -> w16
        tunnel: w13 -> [w84]
        tunnel: [w84] -> w12
        tunnel: w4 -> [w82]
        tunnel: w10 -> [w94]
        tunnel: w20 -> [w99]
        tunnel: w19 -> [w104]
        tunnel: w18 -> [w102]
        tunnel: w17 -> [w101]
        tunnel: w16 -> [w100]
        tunnel: [w100] -> w15
        tunnel: w12 -> [w96]
        tunnel: w15 -> [w122]
        frame #0 {
          n44 = disable-structure shown="Enabled" {
            disable-tunnel: w83 -> [w90 w91]
            disable-tunnel: w82 -> [w89 _]
            disable-tunnel: [w88 w91] -> w79
            frame Enabled {
              n45 = Multiply(x=w89, y=w90) -> (x*y=w88:dbl[][])
            }
            frame Disabled {
            }
          }
          "Z 2" <- w79
          n46 = Tick Count (ms)() -> (millisecond timer value=w85:u32)
          n47 = Array Size(array=w82) -> (size(s)=→"size(s)":i32[])
          n48 = Array Size(array=w83) -> (size(s)=→"size(s) 2":i32[])
        }
        frame #1 {
          n49 = Multiply(x=w102, y=w101) -> (x*y=w98:dbl[][])
          n50 = for {
            tunnel: w98 -> [w116] mode=indexing
            tunnel: [w120] -> w105 mode=indexing
            tunnel: w96 -> [w117]
            tunnel: w94 -> [w115]
            tunnel: [w114] -> w97 mode=indexing
            n51 = Multiply(x=w117, y=w116) -> (x*y=w119:dbl[])
            n52 = Divide(x=w116, y=w115) -> (x/y=w114:dbl[])
            n53 = Divide(x=w119, y=w115) -> (x/y=w118:dbl[])
            n54 = Add Array Elements(numeric array=w118) -> (sum=w120:dbl)
          }
          "Array" <- w97
          n55 = Transpose 2D Array(2D array=w98) -> (transposed array=w111:dbl[][])
          n56 = for {
            tunnel: w111 -> [w112] mode=indexing
            tunnel: [w113] -> w108 mode=indexing
            n57 = Add Array Elements(numeric array=w112) -> (sum=w113:dbl)
          }
          n58 = Index Array(array=w99) -> (element=w109:dbl[])  [unwired: 2 in]
          n59 = Bundle("xi"=w109, w108) -> (→"spec cluster 2":cluster{"xi":dbl[], dbl[]})  [unwired: 1 in]
          n60 = call-poly <vilib>:"Numeric Integration.vi"("dt"=w96, "Input Array"=w108) -> ("result"=→"charge (spectra)":dbl)  [unwired: 1 in, 1 out]
          n61 = Bundle("angle (Y)"=w104, w105) -> (→"Sum Y":cluster{"angle (Y)":dbl[], dbl[]})  [unwired: 1 in]
          n62 = call-poly <vilib>:"Numeric Integration.vi"("dt"=w94, "Input Array"=w105) -> ("result"=→"charge (YSum)":dbl)  [unwired: 1 in, 1 out]
          n63 = Multiply(x=w97, y=w96) -> (x*y=w95:dbl[][])
          n64 = Multiply(x=w95, y=w94) -> (x*y=w93:dbl[][])
          "charge density" <- w93
          n65 = Add Array Elements(numeric array=w93) -> (sum=→"charge (sum)":dbl)
        }
        frame #2 {
          n66 = Tick Count (ms)() -> (millisecond timer value=w123:u32)
          n67 = Subtract(x=w123, y=w122) -> (x-y=→"time: spectra":u32)
        }
      }
    }
    frame #2 {
      n68 = Tick Count (ms)() -> (millisecond timer value=w192:u32)
      n69 = Subtract(x=w192, y=w191) -> (x-y=→"time: 2Dinter":u32)
    }
  }
